vi "Swerve Post (1).vi"(4 "reverse encoder":bool=TRUE, 5 "reverse steer":bool=TRUE, 6 "gear ratio":dbl, 7 "ScaleSpeed":dbl, 9 "wa in":dbl, 10 "ws in":dbl, 11 "encoder in":i32) -> (1 "wa out":dbl, 2 "ws out 0-1":dbl)   [LabVIEW 2020]
panel:
  out "wa (new)":dbl
  out "encoder fraction":dbl
  out "encoder int":dbl
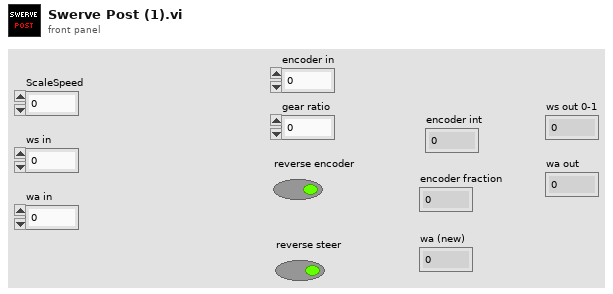
[diagram p1: front panel]
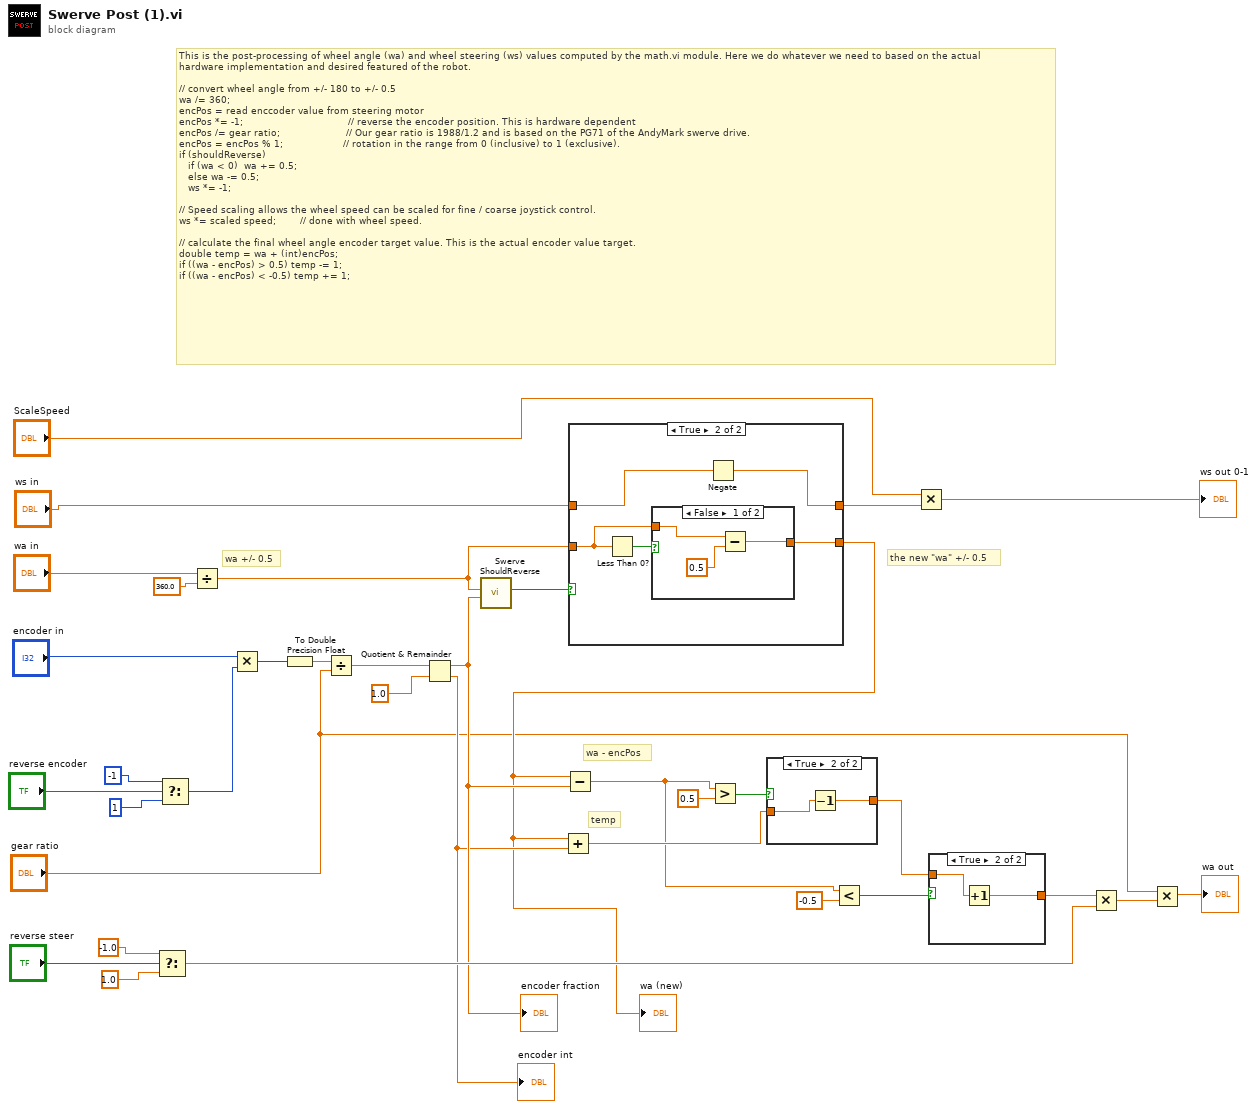
[diagram p0: block diagram]
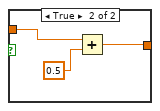
[diagram p5: hidden frame]
diagram:
  # "wa - encPos"
  # "temp"
  # "the new \"wa\" +/- 0.5"
  # "wa +/- 0.5"
  # "This is the post-processing of wheel angle (wa) and wheel steering (ws) values computed by the math.vi module. Here we do whatever we need to based on the actual\nhardware implementation and desired featured of the robot.\n\n// convert wheel angle from +/- 180 to +/- 0.5\nwa /= 360;\nencPos = read enccoder value from steering motor\nencPos *= -1;                                   // reverse the encoder position. This is hardware dependent\nencPos /= gear ratio;                      // Our gear ratio is 1988/1.2 and is based on the PG71 of the AndyMark swerve drive.\nencPos = encPos % 1;                    // rotation in the range from 0 (inclusive) to 1 (exclusive). \nif (shouldReverse)\n   if (wa < 0)  wa += 0.5;\n   else wa -= 0.5;\n   ws *= -1;\n\n// Speed scaling allows the wheel speed can be scaled for fine / coarse joystick control.\nws *= scaled speed;        // done with wheel speed.\n\n// calculate the final wheel angle encoder target value. This is the actual encoder value target.\ndouble temp = wa + (int)encPos;\nif ((wa - encPos) > 0.5) temp -= 1;\nif ((wa - encPos) < -0.5) temp += 1;"
  n1 = Select(t=-1.0, s="reverse steer", f=1.0) -> (s? t:f=w8:dbl)
  n2 = Select(t=-1, s="reverse encoder", f=1) -> (s? t:f=w27:i32)
  n3 = Divide(x="wa in", y=360.0) -> (x/y=w24:dbl)
  n4 = Multiply(x="encoder in", y=w27) -> (x*y=w26:i32)
  n5 = To Double Precision Float(number=w26) -> (double precision float=w25:dbl)
  n6 = Divide(x=w25, y="gear ratio") -> (x/y=w34:dbl)
  n7 = Quotient & Remainder(x=w34, y=1.0) -> (x-y*floor(x/y)=w7:dbl, floor(x/y)=w6:dbl)
  "encoder int" <- w6
  "encoder fraction" <- w7
  n8 = call "Swerve ShouldReverse.vi"("ca in"=w7, "wa in"=w24) -> ("shouldReverse out"=w31:bool)  [unwired: 9 in]
  n9 = case shown="True" w31 {
    tunnel: "ws in" -> [w37 w38]
    tunnel: w24 -> [w36 w41]
    tunnel: [w37 w39] -> w23
    tunnel: [w36 w40] -> w5
    frame False {
    }
    frame True {
      n10 = Less Than 0?(x=w41) -> (x < 0?=w42:bool)
      n11 = case shown="False" w42 {
        tunnel: w41 -> [w44 w47]
        tunnel: [w43 w46] -> w40
        frame False {
          n12 = Subtract(x=w44, y=0.5) -> (x-y=w43:dbl)
        }
        frame True {
          n13 = Add(x=w47, y=0.5) -> (x+y=w46:dbl)
        }
      }
      n14 = Negate(x=w38) -> (-x=w39:dbl)
    }
  }
  "wa (new)" <- w5
  n15 = Add(x=w5, y=w6) -> (x+y=w17:dbl)
  n16 = Subtract(x=w5, y=w7) -> (x-y=w14:dbl)
  n17 = Greater?(x=w14, y=0.5) -> (0:w18:bool)
  n18 = case shown="True" w18 {
    tunnel: w17 -> [w49 w51]
    tunnel: [w49 w50] -> w13
    frame False {
    }
    frame True {
      n19 = Decrement(x=w51) -> (x-1=w50:dbl)
    }
  }
  n20 = Less?(x=w14, y=-0.5) -> (x < y?=w16:bool)
  n21 = Multiply(x="ScaleSpeed", y=w23) -> (x*y=→"ws out 0-1":dbl)
  n22 = case shown="True" w16 {
    tunnel: w13 -> [w52 w54]
    tunnel: [w52 w53] -> w12
    frame False {
    }
    frame True {
      n23 = Increment(x=w54) -> (x+1=w53:dbl)
    }
  }
  n24 = Multiply(x=w12, y=w8) -> (x*y=w4:dbl)
  n25 = Multiply(x="gear ratio", y=w4) -> (x*y=→"wa out":dbl)
